vi "Clean Subscriptions.vi"(10 "Subscriptions in":refnum<class "Subscription.lvclass">[](array[class])) -> (2 "Subscriptions":refnum<class "Subscription.lvclass">[](array[class]))   [LabVIEW 2013, in "MQTT Base.lvlib" / "MQTT_Base.lvclass"]
uses:
  MQTT_Base.lvclass
  Subscription/Subscription.lvclass
  Subscription/Subscription.lvclass/Subscription.ctl
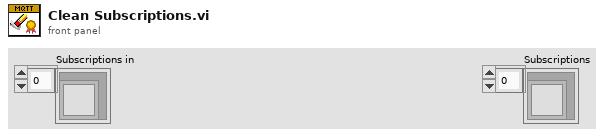
[diagram p1: front panel]
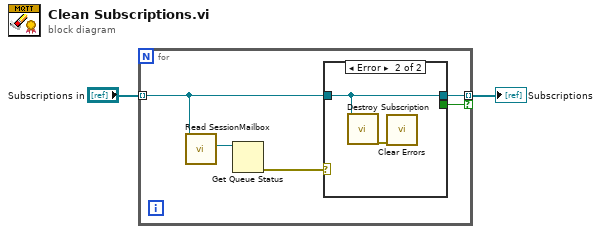
[diagram p0: block diagram]
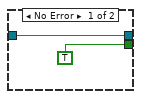
[diagram p2: hidden frame]
diagram:
  n1 = for {
    tunnel: "Subscriptions in" -> [w4] mode=indexing
    tunnel: [w5] -> w1 mode=indexing if=w3
    n2 = call "Read SessionMailbox.vi"("Subscription in"=w4) -> ("SessionMailbox"=w7:refnum<queue>)  [unwired: 8 in, 2 out]
    n3 = Get Queue Status(queue=w7) -> (error out=w6:errorcluster)  [unwired: 2 in, 7 out]
    n4 = case shown="Error" w6 {
      tunnel: [w9 w11] -> w5
      tunnel: w4 -> [w9 w11]
      tunnel: [TRUE _] -> w3
      frame No Error {
      }
      frame Error {
        n5 = call "Destroy Subscription.vi"("Subscription in"=w11) -> ("error out"=w10:errorcluster)  [unwired: 9 in, 1 out]
        n6 = call <vilib>:"Clear Errors.vi"("error in (no error)"=w10) -> ()  [unwired: 6 in, 1 out]
      }
    }
  }
  "Subscriptions" <- w1
